vi "myOptionUI.vi"(8 "响应(2号)端口类型":u8(ring)=2 items=["单相", "三相αβ系", "三相同步系", "三相正负序"], 9 "注入(1号)端口类型":u8(ring)=2 items=["单相", "三相αβ系", "三相同步系", "三相正负序"], 10 "同步相位来源":u8(ring) items=["1号A相", "2号A相"], 11 "测量模式":u8(ring)=2 items=["仅测量信号", "扫频"]) -> (0 "频点预览模式":u8, 1 "if 需要设置触发":bool, 2 "同步相位来源结果":u8, 3 "if 显示同步相位选项":bool, 4 "csv中存储列分别为":string, 5 "需要的示波器台数":u8, 6 "测试选项说明":string, 7 "if 显示端口类型选项":bool)   [LabVIEW 2024]
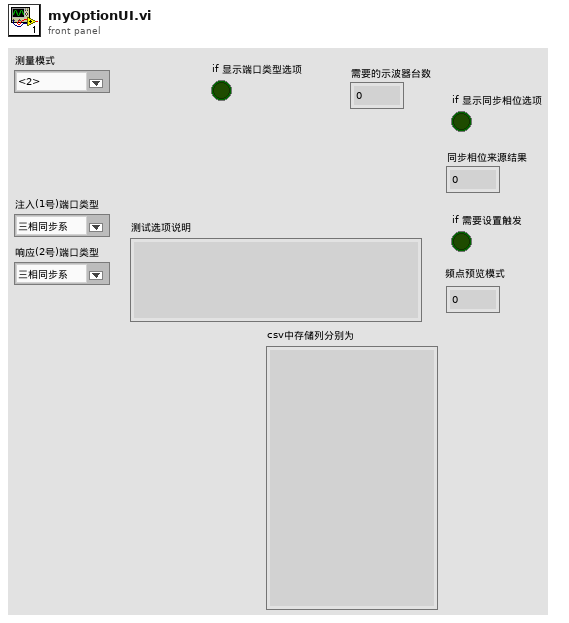
[diagram p1: front panel]
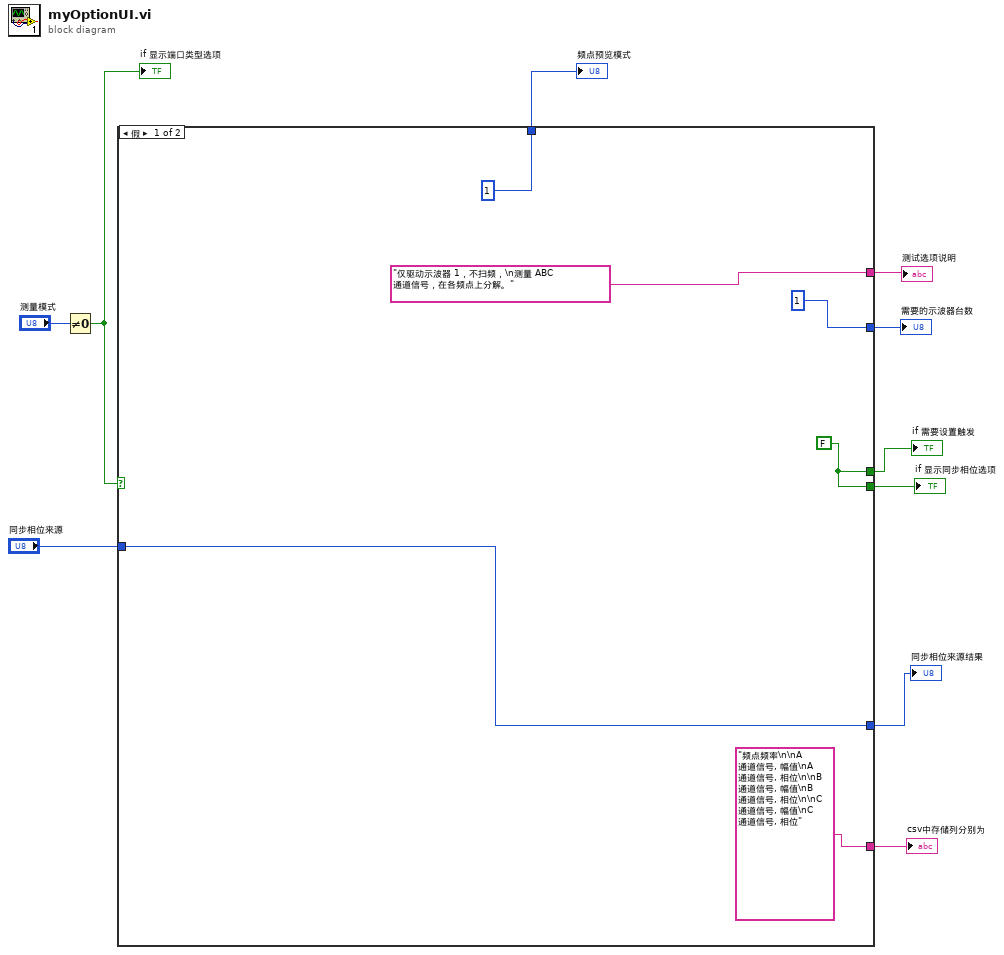
[diagram p0: block diagram]
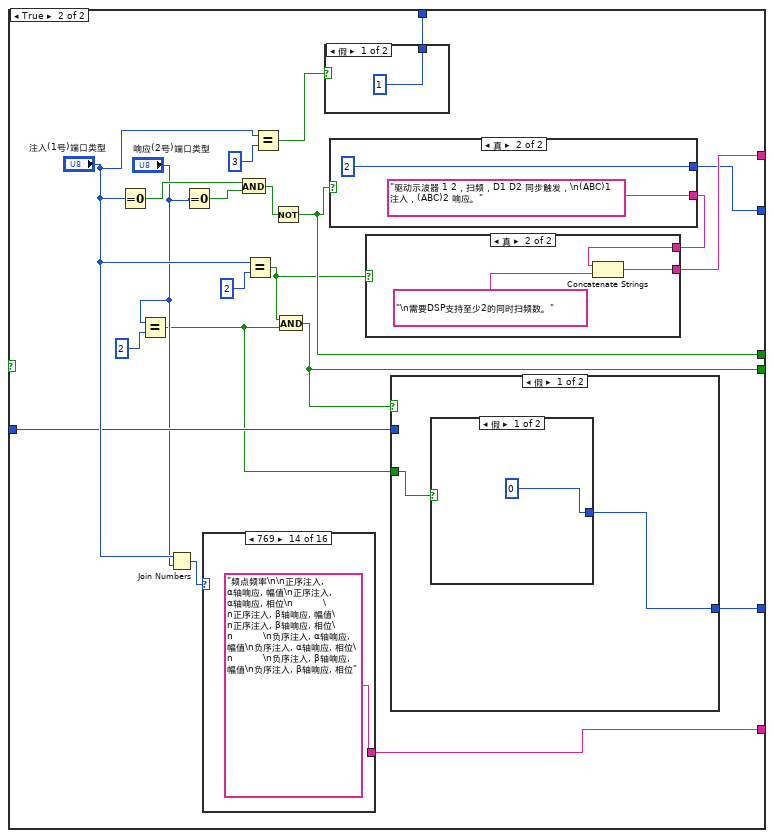
[diagram p2: hidden frame]
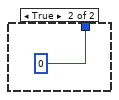
[diagram p3: hidden frame]
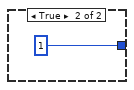
[diagram p4: hidden frame]
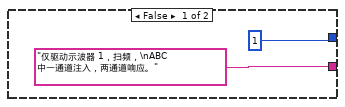
[diagram p7: hidden frame]
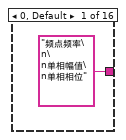
[diagram p8: hidden frame]
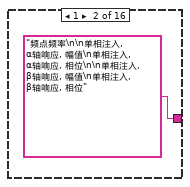
[diagram p9: hidden frame]
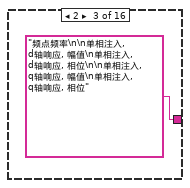
[diagram p10: hidden frame]
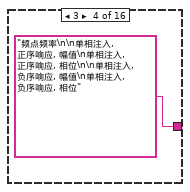
[diagram p11: hidden frame]
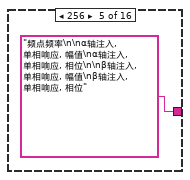
[diagram p12: hidden frame]
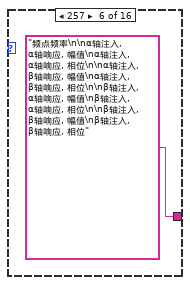
[diagram p13: hidden frame]
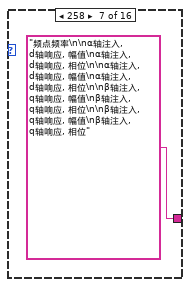
[diagram p14: hidden frame]
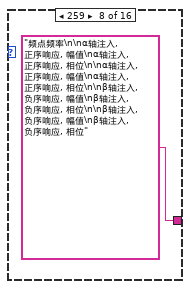
[diagram p15: hidden frame]
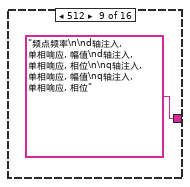
[diagram p16: hidden frame]
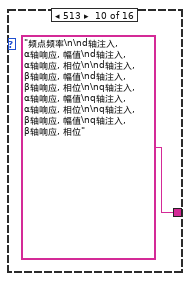
[diagram p17: hidden frame]
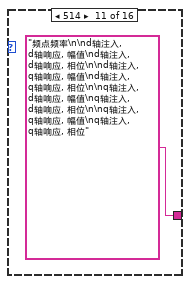
[diagram p18: hidden frame]
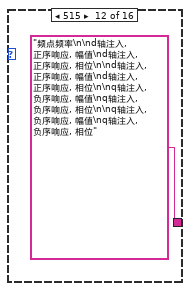
[diagram p19: hidden frame]
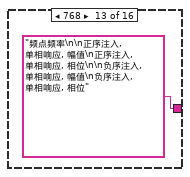
[diagram p20: hidden frame]
diagram:
  n1 = Not Equal To 0?(x="测量模式") -> (x != 0?=w9:bool)
  "if 显示端口类型选项" <- w9
  n2 = case shown="假" w9 {
    tunnel: ["频点频率\n\nA 通道信号, 幅值\nA 通道信号, 相位\n\nB 通道信号, 幅值\nB 通道信号, 相位\n\nC 通道信号, 幅值\nC 通道信号, 相位" w36] -> w8
    tunnel: ["仅驱动示波器 1，不扫频，\n测量 ABC 通道信号，在各频点上分解。" w31] -> w7
    tunnel: [w13 w29] -> w6
    tunnel: [u8 1 w28] -> w5
    tunnel: [w13 w24] -> w4
    tunnel: "同步相位来源" -> [w12 w22]
    tunnel: [w12 w23] -> w2
    tunnel: [u8 1 w17] -> w1
    frame False {
      w13 = FALSE
    }
    frame True {
      n3 = Equal To 0?(x="注入(1号)端口类型") -> (x = 0?=w35:bool)
      n4 = Equal?(x="响应(2号)端口类型", y=u8 2) -> (x = y?=w19:bool)
      n5 = Join Numbers(hi="注入(1号)端口类型", lo="响应(2号)端口类型") -> ((hi.lo)=w37:u16)
      n6 = Equal To 0?(x="响应(2号)端口类型") -> (x = 0?=w34:bool)
      n7 = case shown="769" w37 {
        tunnel: ["频点频率\n\n单相幅值\n单相相位" "频点频率\n\n单相注入, α轴响应, 幅值\n单相注入, α轴响应, 相位\n\n单相注入, β轴响应, 幅值\n单相注入, β轴响应, 相位" "频点频率\n\n单相注入, d轴响应, 幅值\n单相注入, d轴响应, 相位\n\n单相注入, q轴响应, 幅值\n单相注入, q轴响应, 相位" "频点频率\n\n单相注入, 正序响应, 幅值\n单相注入, 正序响应, 相位\n\n单相注入, 负序响应, 幅值\n单相注入, 负序响应, 相位" "频点频率\n\nα轴注入, 单相响应, 幅值\nα轴注入, 单相响应, 相位\n\nβ轴注入, 单相响应, 幅值\nβ轴注入, 单相响应, 相位" "频点频率\n\nα轴注入, α轴响应, 幅值\nα轴注入, α轴响应, 相位\n\nα轴注入, β轴响应, 幅值\nα轴注入, β轴响应, 相位\n\nβ轴注入, α轴响应, 幅值\nβ轴注入, α轴响应, 相位\n\nβ轴注入, β轴响应, 幅值\nβ轴注入, β轴响应, 相位" "频点频率\n\nα轴注入, d轴响应, 幅值\nα轴注入, d轴响应, 相位\n\nα轴注入, d轴响应, 幅值\nα轴注入, d轴响应, 相位\n\nβ轴注入, q轴响应, 幅值\nβ轴注入, q轴响应, 相位\n\nβ轴注入, q轴响应, 幅值\nβ轴注入, q轴响应, 相位" "频点频率\n\nα轴注入, 正序响应, 幅值\nα轴注入, 正序响应, 相位\n\nα轴注入, 正序响应, 幅值\nα轴注入, 正序响应, 相位\n\nβ轴注入, 负序响应, 幅值\nβ轴注入, 负序响应, 相位\n\nβ轴注入, 负序响应, 幅值\nβ轴注入, 负序响应, 相位" "频点频率\n\nd轴注入, 单相响应, 幅值\nd轴注入, 单相响应, 相位\n\nq轴注入, 单相响应, 幅值\nq轴注入, 单相响应, 相位" "频点频率\n\nd轴注入, α轴响应, 幅值\nd轴注入, α轴响应, 相位\n\nd轴注入, β轴响应, 幅值\nd轴注入, β轴响应, 相位\n\nq轴注入, α轴响应, 幅值\nq轴注入, α轴响应, 相位\n\nq轴注入, β轴响应, 幅值\nq轴注入, β轴响应, 相位" "频点频率\n\nd轴注入, d轴响应, 幅值\nd轴注入, d轴响应, 相位\n\nd轴注入, q轴响应, 幅值\nd轴注入, q轴响应, 相位\n\nq轴注入, d轴响应, 幅值\nq轴注入, d轴响应, 相位\n\nq轴注入, q轴响应, 幅值\nq轴注入, q轴响应, 相位" "频点频率\n\nd轴注入, 正序响应, 幅值\nd轴注入, 正序响应, 相位\n\nd轴注入, 正序响应, 幅值\nd轴注入, 正序响应, 相位\n\nq轴注入, 负序响应, 幅值\nq轴注入, 负序响应, 相位\n\nq轴注入, 负序响应, 幅值\nq轴注入, 负序响应, 相位" "频点频率\n\n正序注入, 单相响应, 幅值\n正序注入, 单相响应, 相位\n\n负序注入, 单相响应, 幅值\n负序注入, 单相响应, 相位" "频点频率\n\n正序注入, α轴响应, 幅值\n正序注入, α轴响应, 相位\n          \n正序注入, β轴响应, 幅值\n正序注入, β轴响应, 相位\n          \n负序注入, α轴响应, 幅值\n负序注入, α轴响应, 相位\n          \n负序注入, β轴响应, 幅值\n负序注入, β轴响应, 相位" "频点频率\n\n正序注入, d轴响应, 幅值\n正序注入, d轴响应, 相位\n          \n正序注入, q轴响应, 幅值\n正序注入, q轴响应, 相位\n          \n负序注入, d轴响应, 幅值\n负序注入, d轴响应, 相位\n          \n负序注入, q轴响应, 幅值\n负序注入, q轴响应, 相位" "频点频率\n\n正序注入, 正序响应, 幅值\n正序注入, 正序响应, 相位\n\n正序注入, 负序响应, 幅值\n正序注入, 负序响应, 相位\n\n负序注入, 正序响应, 幅值\n负序注入, 正序响应, 相位\n\n负序注入, 负序响应, 幅值\n负序注入, 负序响应, 相位"] -> w36
        frame 0, Default {
        }
        frame 1 {
        }
        frame 2 {
        }
        frame 3 {
        }
        frame 256 {
        }
        frame 257 {
        }
        frame 258 {
        }
        frame 259 {
        }
        frame 512 {
        }
        frame 513 {
        }
        frame 514 {
        }
        frame 515 {
        }
        frame 768 {
        }
        frame 769 {
        }
        frame 770 {
        }
        frame 771 {
        }
      }
      n8 = And(x=w35, y=w34) -> (x .and. y?=w30:bool)
      n9 = Equal?(x="注入(1号)端口类型", y=u8 2) -> (x = y?=w21:bool)
      n10 = Equal?(x="注入(1号)端口类型", y=u8 3) -> (x = y?=w18:bool)
      n11 = Not(x=w30) -> (.not. x?=w29:bool)
      n12 = And(x=w21, y=w19) -> (x .and. y?=w24:bool)
      n13 = case shown="假" w18 {
        tunnel: [u8 1 u8 0] -> w17
        frame False {
        }
        frame True {
        }
      }
      n14 = case shown="真" w29 {
        tunnel: ["仅驱动示波器 1，扫频，\nABC 中一通道注入，两通道响应。" "驱动示波器 1 2，扫频，D1 D2 同步触发，\n(ABC)1 注入，(ABC)2 响应。"] -> w32
        tunnel: [u8 1 u8 2] -> w28
        frame False {
        }
        frame True {
        }
      }
      n15 = case shown="真" w21 {
        tunnel: w32 -> [w45 w47]
        tunnel: [w45 w46] -> w31
        frame False {
        }
        frame True {
          n16 = Concatenate Strings(w47, "\n需要DSP支持至少2的同时扫频数。") -> (w46:string)
        }
      }
      n17 = case shown="假" w24 {
        tunnel: [w40 w44] -> w23
        tunnel: w22 -> [_ w44]
        tunnel: w19 -> [w41 _]
        frame False {
          n18 = case shown="假" w41 {
            tunnel: [u8 0 u8 1] -> w40
            frame False {
            }
            frame True {
            }
          }
        }
        frame True {
        }
      }
    }
  }
  "if 显示同步相位选项" <- w4
  "同步相位来源结果" <- w2
  "if 需要设置触发" <- w6
  "频点预览模式" <- w1
  "测试选项说明" <- w7
  "csv中存储列分别为" <- w8
  "需要的示波器台数" <- w5
